vi "LabVIEW Simulator MAIN.vi"() -> ()   [LabVIEW 2018]
panel:
  out "restarted 2":bool
  out "restarted":bool
  out "pulse_per_volume":dbl=1.0
  out "Tplateau":dbl=150.0
  out "Psex":dbl
  out "Psin":dbl
  out "Vex":dbl
  out "Vin":dbl
  out "Tex":dbl
  out "Tin":dbl
  out "T":dbl
  out "plateau pressure":i32
  out "pressure":i32
  out "start":bool=TRUE
  out "peep":i32
  in  "VT":i32
  out "PIN_LED 13":bool
  out "PIN_MOTOR_STEP_ORIGIN 12":bool
  out "PIN_MOTOR_STEP_FORTH 11":bool
  out "PIN_BUZZER 9":bool
  out "PIN_MOTOR_STEP_BACK 10":bool
  in  "PIN_INP 7":bool
  in  "PIN_SETON 6":bool
  in  "PIN_BUSY 5":bool
  in  "PIN_WAREA 4":bool
  in  "PIN_SWITCH_ERR_ACK 3":bool
  in  "PIN_SWITCH_ONOFF 2":bool
  in  "PIN_PRESSURE_IN A3":dbl(slide) scale=0.0..1024.0
  in  "PIN_PEEP_IN A3":dbl(knob) scale=0.0..1024.0
  in  "PIN_IE_IN A2":dbl(knob) scale=0.0..1024.0
  in  "PIN_VT_IN A1":dbl(knob) scale=0.0..1024.0
  in  "PIN_BPM_IN A0":dbl(knob) scale=0.0..1024.0
  # "GEVE Emergency Medical Ventilator Simulation"
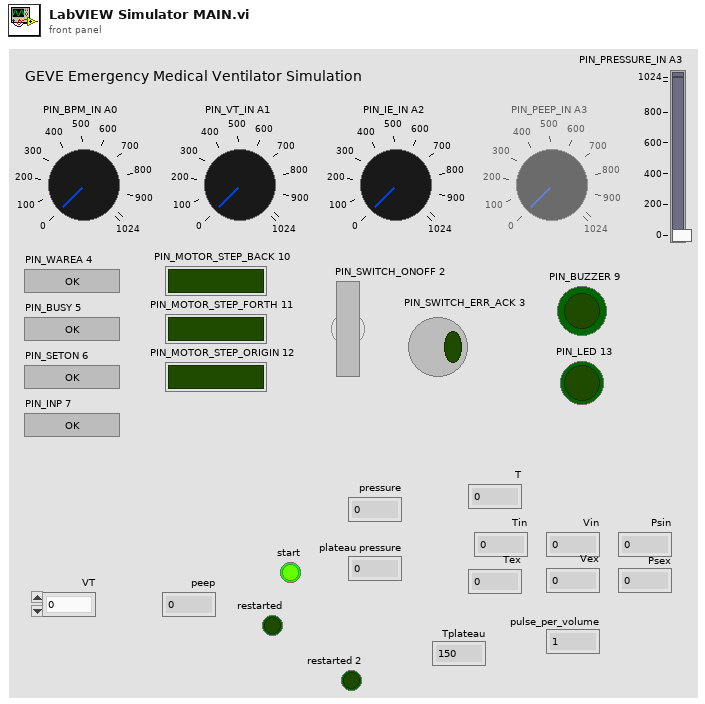
[diagram p1: front panel]
types:
  T1 = enum16{"STOP", "SET_INIT", "INIT", "SET_INHALE", "INHALE", "SET_PAUSE", "PAUSE", "SET_EXHALE", "EXHALE"}
  T2 = enum16{"STATE_OK", "STATE_ERR_HIGH_PRESSURE", "STATE_ERR_LOW_PRESSURE", "STATE_ERR_FAIL_INIT", "STATE_ERR_MOTOR"}
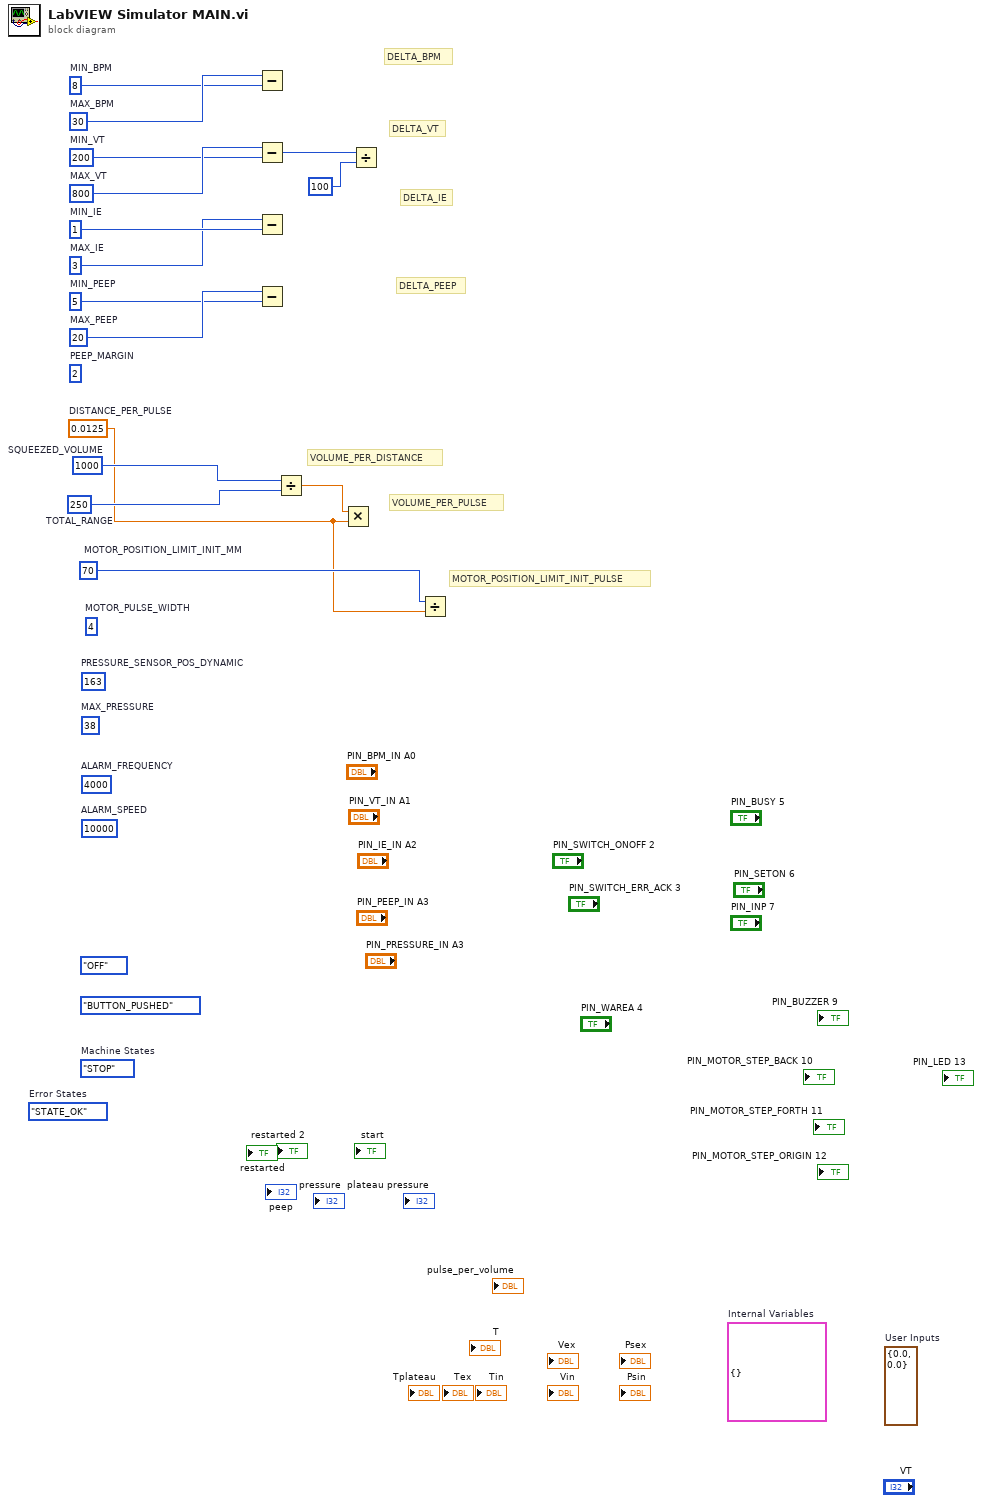
[diagram p0: block diagram]
diagram:
  (unwired) cluster{"bpm":dbl, "IE":dbl} {"bpm"=0.0, "IE"=0.0}  # User Inputs
  (unwired) cluster{} {}  # Internal Variables
  (unwired) T1."STOP"  # Machine States
  (unwired) enum16{"BUTTON_PUSHED", "BUTTON_RELEASED"}."BUTTON_PUSHED"
  (unwired) enum16{"OFF", "ON"}."OFF"
  (unwired) T2."STATE_OK"  # Error States
  (unwired) 10000  # ALARM_SPEED
  (unwired) 4000  # ALARM_FREQUENCY
  (unwired) 38  # MAX_PRESSURE
  (unwired) 163  # PRESSURE_SENSOR_POS_DYNAMIC
  (unwired) 4  # MOTOR_PULSE_WIDTH
  w2 = 70  # MOTOR_POSITION_LIMIT_INIT_MM
  w4 = 250  # TOTAL_RANGE
  w5 = 1000  # SQUEEZED_VOLUME
  w1 = 0.0125  # DISTANCE_PER_PULSE
  (unwired) 2  # PEEP_MARGIN
  w7 = 20  # MAX_PEEP
  w6 = 5  # MIN_PEEP
  w8 = 3  # MAX_IE
  w9 = 1  # MIN_IE
  w15 = 800  # MAX_VT
  w14 = 200  # MIN_VT
  w13 = 30  # MAX_BPM
  w12 = 8  # MIN_BPM
  # "MOTOR_POSITION_LIMIT_INIT_PULSE"
  # "VOLUME_PER_PULSE"
  # "VOLUME_PER_DISTANCE"
  # "DELTA_PEEP"
  # "DELTA_IE"
  # "DELTA_VT"
  # "DELTA_BPM"
  n1 = Subtract(x=w13, y=w12) -> ()  [unwired: 1 out]
  n2 = Subtract(x=w15, y=w14) -> (x-y=w11:i32)
  n3 = Subtract(x=w8, y=w9) -> ()  [unwired: 1 out]
  n4 = Subtract(x=w7, y=w6) -> ()  [unwired: 1 out]
  n5 = Divide(x=w5, y=w4) -> (x/y=w3:dbl)
  n6 = Multiply(x=w3, y=w1) -> ()  [unwired: 1 out]
  n7 = Divide(x=w11, y=100) -> ()  [unwired: 1 out]
  n8 = Divide(x=w2, y=w1) -> ()  [unwired: 1 out]
